vi "Read Masked SSL Protocols.vi"(8 "error in (no error)":errorcluster, 11 "dotNET SSL Socket in":refnum<class "dotNET SSL Socket.lvclass">) -> (0 "error out":errorcluster, 2 "Masked SSL Protocols":i32, 3 "dotNET SSL Socket out":refnum<class "dotNET SSL Socket.lvclass">)   [LabVIEW 2013, in "dotNET SSL Socket.lvlib" / "dotNET SSL Socket.lvclass"]
uses:
  dotNET SSL Socket.lvclass
  dotNET SSL Socket.lvclass/dotNET SSL Socket.ctl
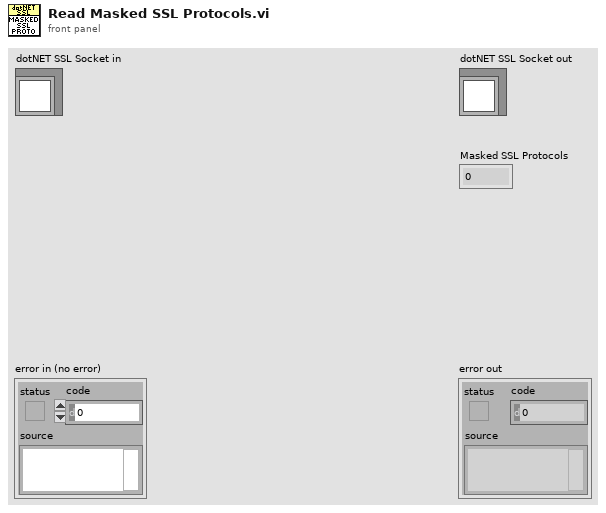
[diagram p1: front panel]
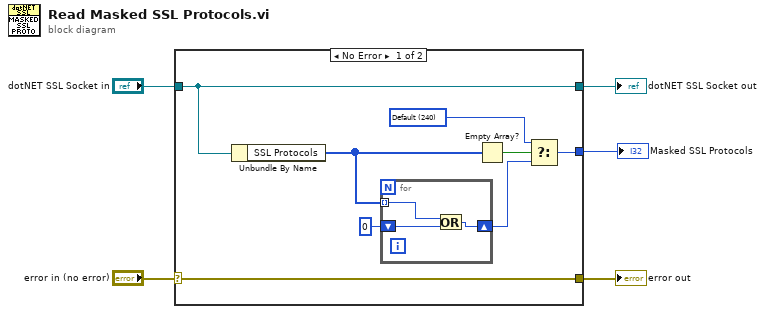
[diagram p0: block diagram]
diagram:
  n1 = case shown="No Error" "error in (no error)" {
    selector: "error in (no error)" -> [w13 w18]
    tunnel: [w13 w18] -> w4
    tunnel: [w12 w17] -> w2
    tunnel: "dotNET SSL Socket in" -> [w12 w17]
    tunnel: [w6 _] -> w1
    frame No Error {
      w8 = 240 items=["None"=0, "Ssl2"=12, "Ssl3"=48, "Tls"=192, "Default"=240, "Tls11"=768, "Tls12"=3072] ("enabledSslProtocols")
      n2 = Unbundle By Name(w12) -> ("SSL Protocols"=w10:i32[])
      n3 = for {
        tunnel: w10 -> [w16] mode=indexing
        shift-right: [w15] -> w7
        shift-left: 0 -> [w14]
        n4 = Or(x=w16, y=w14) -> (x .or. y?=w15:i32)
      }
      n5 = Empty Array?(array=w10) -> (empty?=w9:bool)
      n6 = Select(t=w8, s=w9, f=w7) -> (s? t:f=w6:i32)
    }
    frame Error {
    }
  }
  "error out" <- w4
  "dotNET SSL Socket out" <- w2
  "Masked SSL Protocols" <- w1
